vi "Forebrain Main.vi"(2 "QueueRef":T1, 3 "NotifierReff":T2) -> ()   [LabVIEW 2013]
uses:
  Data/TypeDefs/Notifiers.ctl
  Data/TypeDefs/UTM Location.ctl
  Data/TypeDefs/Sail Set Suggestions.ctl
  Data/TypeDefs/Rudder Set Suggestions.ctl
  Data/TypeDefs/OverrideInformation.ctl
  Data/TypeDefs/OverrideMode.ctl
  Data/TypeDefs/MotorSetup.ctl
  Data/TypeDefs/DynamixelSetupInfo.ctl
  Classes/Missions/GenericMission/GenericMission.lvclass
  Data/TypeDefs/Queues.ctl
  Classes/Waypoint/Waypoint.lvclass
  RIO-OCU_Comm/NetworkStreams/Reader/NetworkStreamReader.lvclass
panel:
  out "MissionArraySize":i32
  in  "stop":bool
  out "UpdatedMissionArray":refnum<class "GenericMission.lvclass">[](array[class])
  in  "error in (no error)":errorcluster
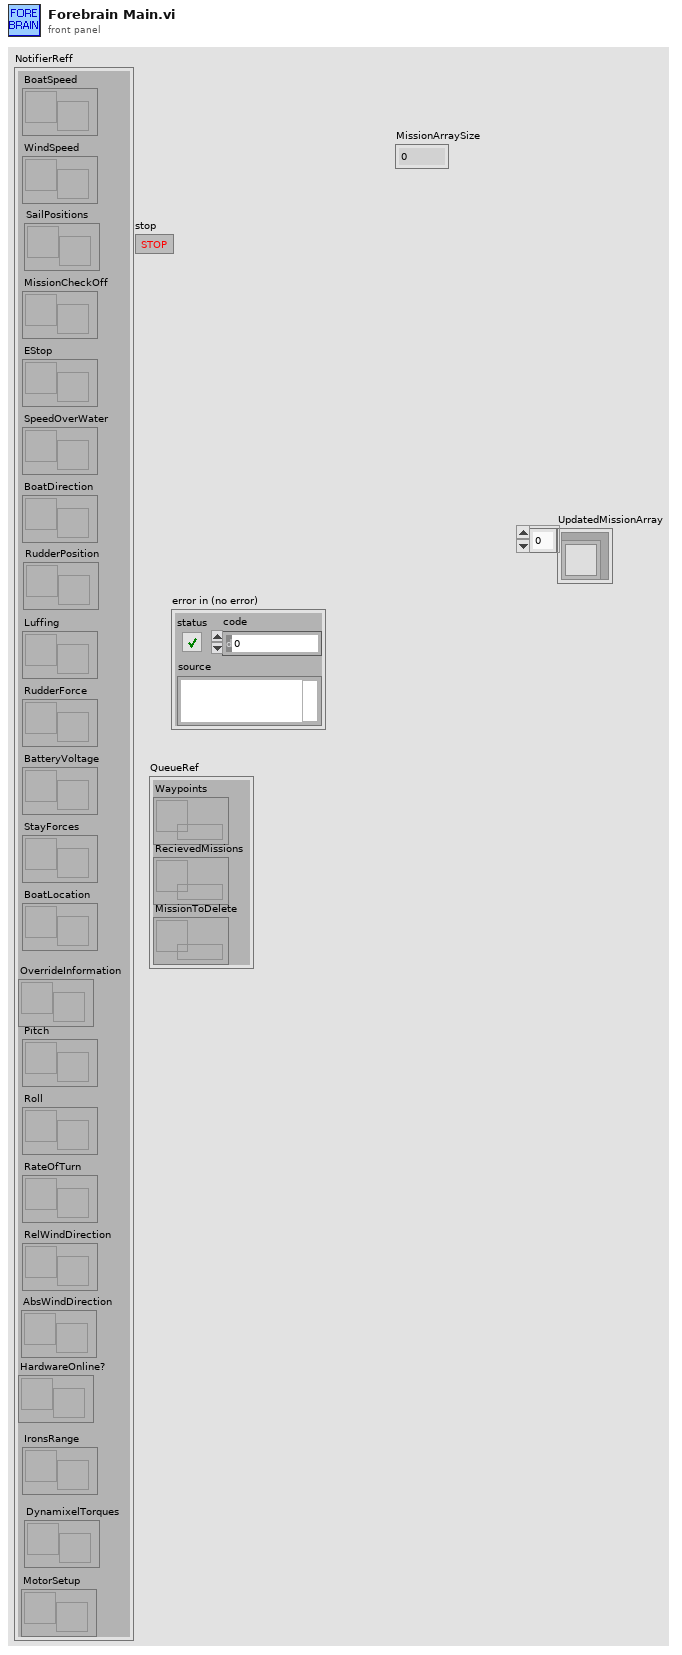
[diagram p1: front panel]
types:
  T1 = typedef "Queues.ctl" = cluster{"Waypoints":refnum<queue>, "RecievedMissions":refnum<queue>, "MissionToDelete":refnum<queue>}
  T2 = typedef "Notifiers.ctl" = cluster{"BoatSpeed":refnum<notifier>, "WindSpeed":refnum<notifier>, "MissionCheckOff":refnum<notifier>, "EStop":refnum<notifier>, "SpeedOverWater":refnum<notifier>, "BoatDirection":refnum<notifier>, "Luffing":refnum<notifier>, "RudderForce":refnum<notifier>, "BatteryVoltage":refnum<notifier>, "StayForces":refnum<notifier>, "BoatLocation":refnum<notifier>, "Pitch":refnum<notifier>, "Roll":refnum<notifier>, "RateOfTurn":refnum<notifier>, "RelWindDirection":refnum<notifier>, "SailPositions":refnum<notifier>, "RudderPosition":refnum<notifier>, "IronsRange":refnum<notifier>, "AbsWindDirection":refnum<notifier>, "OverrideInformation":refnum<notifier>, "DynamixelTorques":refnum<notifier>, "HardwareOnline?":refnum<notifier>, "MotorSetup":refnum<notifier>}
  T3 = typedef "UTM Location.ctl" = cluster{"UTM Zone":dbl, "Hemisphere":enum16{"North", "South"}, "East":dbl, "North":dbl}
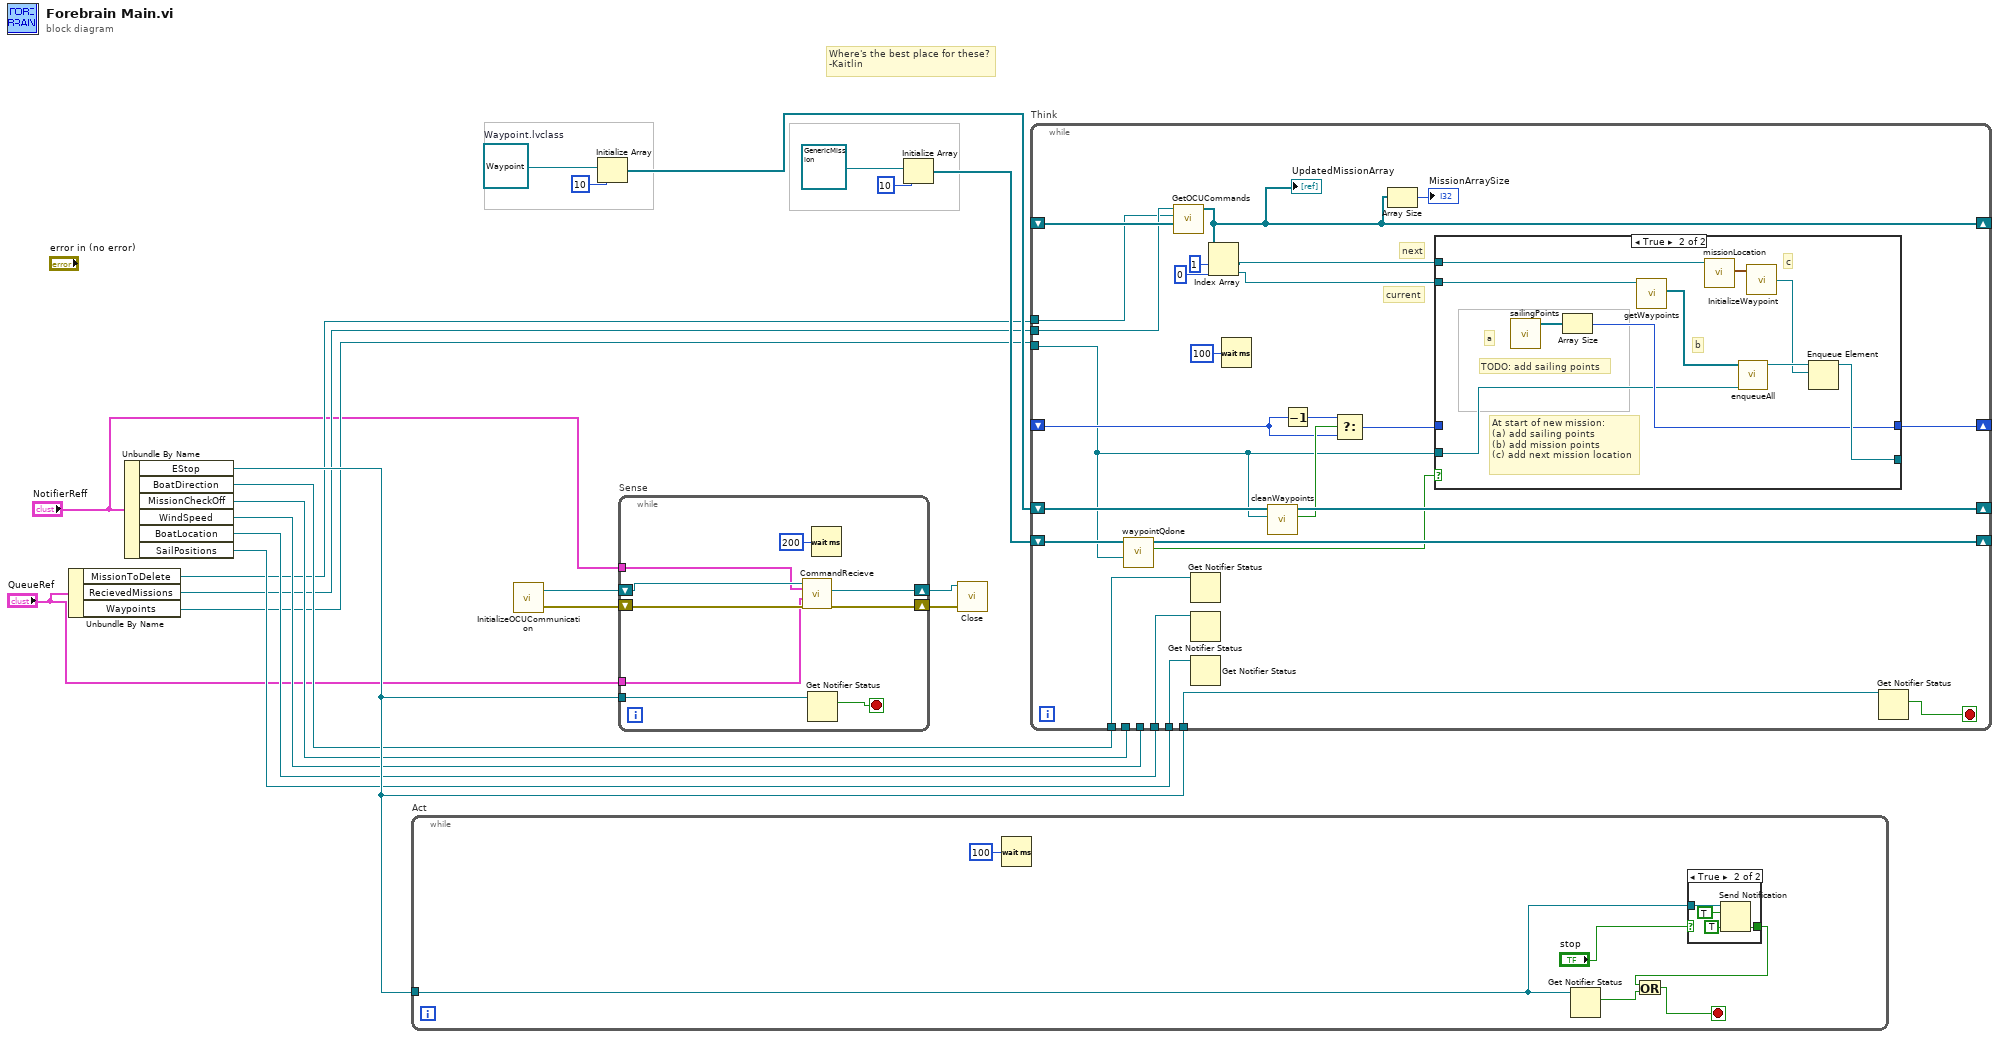
[diagram p0: block diagram]
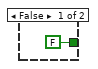
[diagram p2: hidden frame]
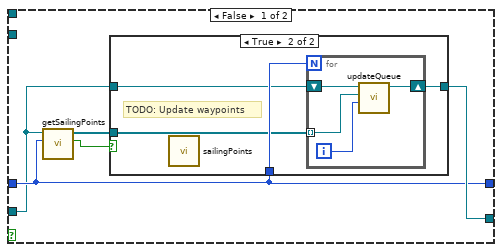
[diagram p3: hidden frame]
diagram:
  w11 = refnum<class "Waypoint.lvclass"> refnum  # Waypoint.lvclass
  # "Where's the best place for these?\n-Kaitlin"
  n1 = Unbundle By Name("QueueRef") -> ("MissionToDelete"=w6:refnum<queue>, "RecievedMissions"=w8:refnum<queue>, "Waypoints"=w9:refnum<queue>)
  n2 = Unbundle By Name("NotifierReff") -> ("EStop"=w21:refnum<notifier>, "BoatDirection"=w20:refnum<notifier>, "MissionCheckOff"=w19:refnum<notifier>, "WindSpeed"=w18:refnum<notifier>, "BoatLocation"=w17:refnum<notifier>, "SailPositions"=w16:refnum<notifier>)
  n3 = while "Act" {
    tunnel: w21 -> [w23]
    stop <- w25 stop-if-true
    n4 = Wait (ms)(milliseconds to wait=u32 100) -> ()  [unwired: 1 out]
    n5 = Get Notifier Status(notifier=w23) -> (current notification=w26:bool)  [unwired: 1 in, 4 out]
    n6 = case shown="True" "stop" {
      tunnel: w23 -> [_ w31]
      tunnel: [FALSE TRUE] -> w22
      frame False {
      }
      frame True {
        n7 = Send Notification(notification=TRUE, notifier=w31) -> ()  [unwired: 1 in, 2 out]
      }
    }
    n8 = Or(x=w22, y=w26) -> (x .or. y?=w25:bool)
  }
  n9 = call "InitializeOCUCommunication.vi"() -> ("error out"=w7:errorcluster, "NetworkStreamWriter out"=w5:refnum<class "NetworkStreamReader.lvclass">)  [unwired: 2 in]
  n10 = Initialize Array(w11, 10 ("dimension size")) -> (w10:refnum<class "Waypoint.lvclass">[])
  n11 = while "Sense" {
    tunnel: w21 -> [w39]
    shift-right: [w37] -> w4
    shift-left: w7 -> [w38]
    shift-right: [w35] -> w3
    shift-left: w5 -> [w34]
    tunnel: "NotifierReff" -> [w33]
    tunnel: "QueueRef" -> [w32]
    stop <- w40 stop-if-true
    n12 = call "CommandRecieve.vi"("error in (no error)"=w38, "input cluster"=w32, "NotifierReff"=w33, "NetworkStreamReader in"=w34) -> ("error out"=w37:errorcluster, "NetworkStreamReader out"=w35:refnum<class "NetworkStreamReader.lvclass">)  [unwired: 6 in]
    n13 = Get Notifier Status(notifier=w39) -> (current notification=w40:bool)  [unwired: 1 in, 4 out]
    n14 = Wait (ms)(milliseconds to wait=u32 200) -> ()  [unwired: 1 out]
  }
  n15 = Initialize Array(refnum<class "GenericMission.lvclass"> refnum ("element"), 10 ("dimension size")) -> (w14:refnum<class "GenericMission.lvclass">[])
  n16 = call "Close.vi"("error in (no error)"=w4, "NetworkStreamReader in"=w3) -> ()  [unwired: 9 in, 1 out]
  n17 = while "Think" {
    tunnel: w20 -> [w60]
    tunnel: w19 -> [_]
    tunnel: w21 -> [w64]
    tunnel: w18 -> [_]
    shift-right: [w42] -> _
    shift-left: _ -> [w59]
    tunnel: w17 -> [w61]
    tunnel: w16 -> [w62]
    shift-right: [w57] -> _
    shift-left: _ -> [w52]
    shift-right: [w56] -> _
    shift-left: w14 -> [w47]
    shift-right: [w66] -> _
    shift-left: w10 -> [w48]
    tunnel: w9 -> [w45]
    tunnel: w8 -> [w46]
    tunnel: w6 -> [w44]
    stop <- w65 stop-if-true
    # "current"
    # "next"
    n18 = call "waypointQdone.vi"("Waypoint Queue"=w45, "Old Missions"=w47) -> ("new mission?"=w55:bool, "Old Missions (updated)"=w56:refnum<class "GenericMission.lvclass">[])  [unwired: 8 in]
    n19 = call "GetOCUCommands.vi"("MissionArray"=w59, "MissionToDelete"=w44, "MissionFromOCU"=w46) -> ("UpdatedMissionArray"=w42:refnum<class "GenericMission.lvclass">[])  [unwired: 7 in, 1 out]
    "UpdatedMissionArray" <- w42
    n20 = Get Notifier Status(notifier=w60) -> ()  [unwired: 1 in, 5 out]
    n21 = Get Notifier Status(notifier=w61) -> ()  [unwired: 1 in, 5 out]
    n22 = Get Notifier Status(notifier=w62) -> ()  [unwired: 1 in, 5 out]
    n23 = Index Array(array=w42, index #1=1 ("index"), index #2=0 ("index")) -> (element #1=w49:refnum<class "GenericMission.lvclass">, element #2=w50:refnum<class "GenericMission.lvclass">)
    n24 = Wait (ms)(milliseconds to wait=u32 100) -> ()  [unwired: 1 out]
    n25 = call "cleanWaypoints.vi"("Waypoint Queue"=w45, "Old Waypoints"=w48) -> ("Done?"=w54:bool, "Old Waypoints (updated)"=w66:refnum<class "Waypoint.lvclass">[])  [unwired: 7 in, 1 out]
    n26 = Decrement(x=w52) -> (x-1=w51:i32)
    n27 = Select(t=w51, s=w54, f=w52) -> (s? t:f=w53:i32)
    n28 = Array Size(array=w42) -> (size(s)=→"MissionArraySize":i32)
    n29 = case shown="True" w55 {
      tunnel: w45 -> [w69 w81]
      tunnel: [w71 w86] -> _
      tunnel: w50 -> [_ w90]
      tunnel: w49 -> [_ w88]
      tunnel: w53 -> [w70 _]
      tunnel: [w70 w82] -> w57
      frame False {
        n30 = call "getSailingPoints.vi"("sailing points left"=w70, "Waypoints"=w69) -> ("remaining sailing points?"=w68:bool, "Array"=w67:refnum<class "Waypoint.lvclass">[])  [unwired: 8 in]
        n31 = case shown="True" w68 {
          tunnel: [w72 w76] -> w71
          tunnel: w70 -> [_ w75]
          tunnel: w69 -> [w72 w74]
          tunnel: w67 -> [_ w73]
          frame False {
          }
          frame True {
            # "TODO: Update waypoints"
            n32 = call "sailingPoints.vi"() -> ()  [unwired: 11 in, 1 out]
            n33 = for {
              N: w75 -> [_]
              shift-right: [w79] -> w76
              shift-left: w74 -> [w80]
              tunnel: w73 -> [w78] mode=indexing
              i -> [w77]
              n34 = call "updateQueue.vi"("Waypoint Index"=w77, "new Waypoint"=w78, "Waypoint Queue"=w80) -> ("queue out"=w79:refnum<queue>)  [unwired: 8 in]
            }
          }
        }
      }
      frame True {
        # "b"
        # "c"
        # "a"
        # "TODO: add sailing points"
        # "At start of new mission:\n(a) add sailing points\n(b) add mission points\n(c) add next mission location"
        n35 = call "sailingPoints.vi"() -> ("Next Sailing Points"=w83:refnum<class "Waypoint.lvclass">[])  [unwired: 11 in]
        n36 = Array Size(array=w83) -> (size(s)=w82:i32)
        n37 = call-dynamic "getWaypoints.vi"("GenericMission in"=w90) -> ("Waypoint Array"=w89:refnum<class "Waypoint.lvclass">[])  [unwired: 8 in, 2 out]
        n38 = call-dynamic "missionLocation.vi"("GenericMission in"=w88) -> ("element"=w85:T3)  [unwired: 8 in, 2 out]
        n39 = call "enqueueAll.vi"("Waypoint Queue"=w81, "Waypoint Array"=w89) -> ("queue out"=w87:refnum<queue>)  [unwired: 9 in]
        n40 = call "InitializeWaypoint.vi"("Coords"=w85) -> ("Waypoint Out"=w84:refnum<class "Waypoint.lvclass">)  [unwired: 2 in]
        n41 = Enqueue Element(queue=w87, element=w84) -> (queue out=w86:refnum<queue>)  [unwired: 2 in, 2 out]
      }
    }
    n42 = Get Notifier Status(notifier=w64) -> (current notification=w65:bool)  [unwired: 1 in, 4 out]
  }
